vi "MB Serial Example Slave.vi"() -> ()   [LabVIEW 2011]
uses:
  MB Slave Init (poly).vi
  MB Globals.vi
  MB Slave Read All Coils (poly).vi
  MB Slave Read All Holding Registers (poly).vi
  MB Slave Write Input Registers (poly).vi
  MB Slave Write Discrete Inputs (poly).vi
panel:
  in  "VISA resource name":refnum<visa-resource-name>
  in  "Slave Address":u8=1 format="%.0x"
  in  "Timeouts":u32[](array[numeric])=[10000]
  in  "Modes":enum16{"RTU", "ASCII"}[](array[ring])=[enum."RTU"]
  in  "Stop":bool
  out "Holding Registers":u16[](array[numeric]) caption="Holding Registers (Master can write in these registers)"
  out "Coils":bool[](array[boolean]) caption="Coils (Master can write coils)"
  in  "Discrete Inputs":bool[](array[boolean])=[FALSE, FALSE, FALSE, FALSE] caption="Discrete Inputs (Master can only read them)"
  in  "Input Registers":u16[](array[numeric])=[0, 0, 0, 0] caption="Input Registers (Master can only read them)"
  # "MB Serial Example Slave.vi\n\nInstructions\n1. Connect your 2 COMs ports using a cross-over cable\n2. Select a COM port in VISA resouce name\n3. Run the VI\n4. Open and run MB Example Master.vi\n5. Modify the discrete inputs or input registers on the slave -> they're updated on the master.\n6. Modify the coils and registers on the master -> they're updated on the slave."
  # "Serial Settings (Other settings imported from MAX)"
  # "Slave Registers"
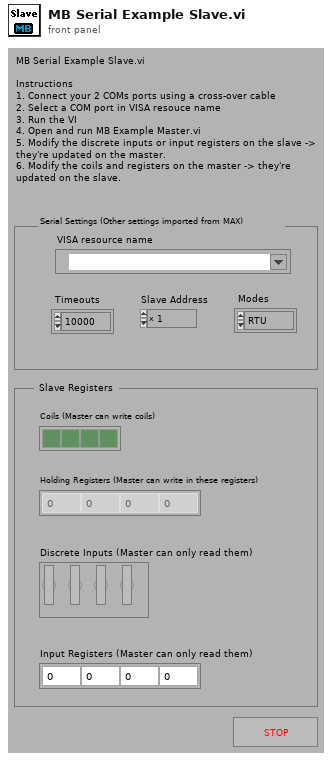
[diagram p1: front panel]
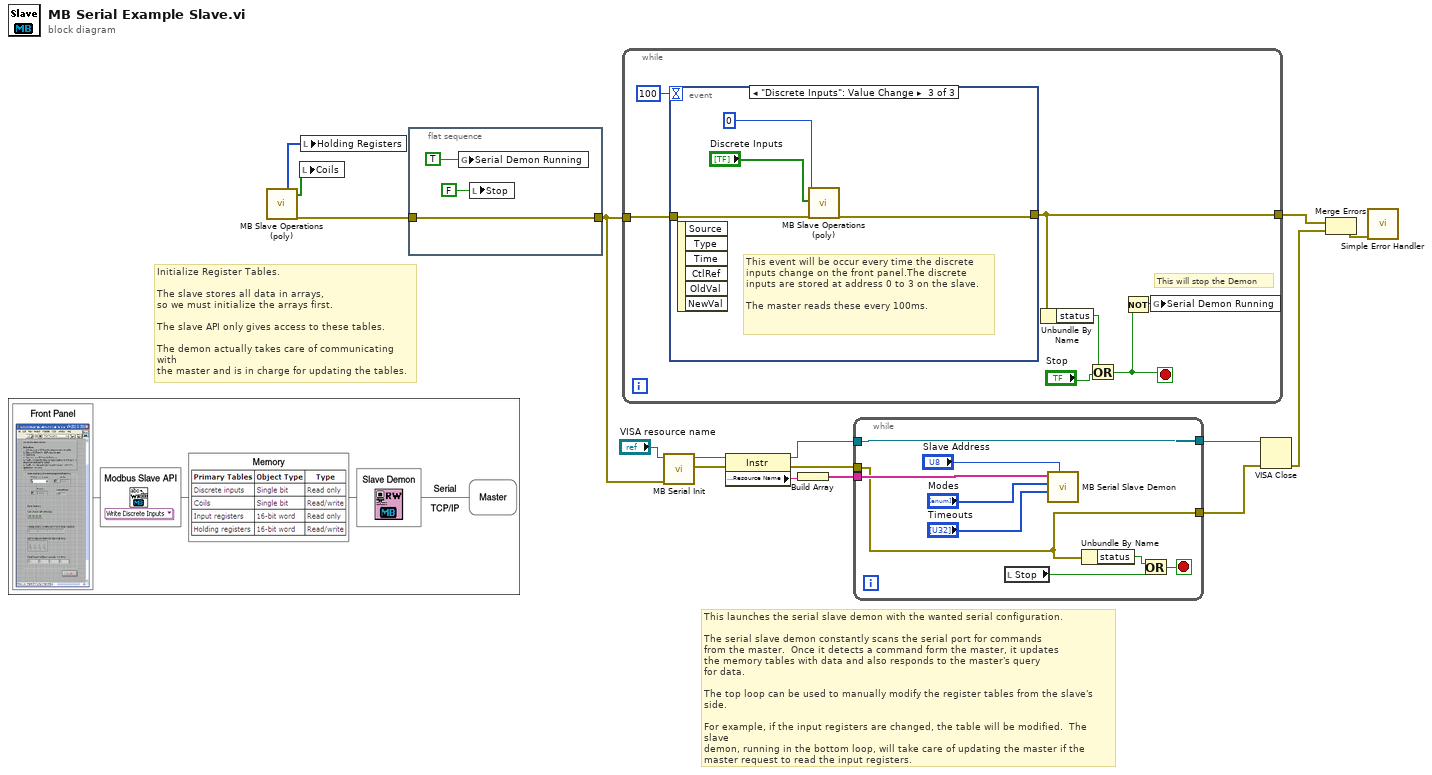
[diagram p0: block diagram]
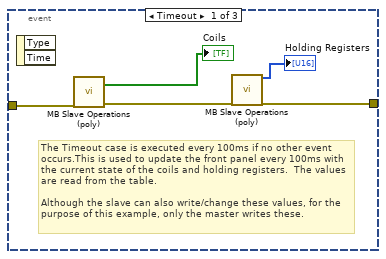
[diagram p2: hidden frame]
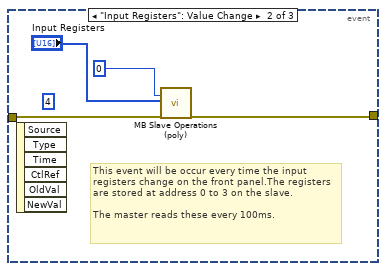
[diagram p3: hidden frame]
diagram:
  # "Initialize Register Tables.\n\nThe slave stores all data in arrays,\nso we must initialize the arrays first.  \n\nThe slave API only gives access to these tables. \n\nThe demon actually takes care of communicating with \nthe master and is in charge for updating the tables."
  # "This launches the serial slave demon with the wanted serial configuration.\n\nThe serial slave demon constantly scans the serial port for commands \nfrom the master.  Once it detects a command form the master, it updates\nthe memory tables with data and also responds to the master's query\nfor data.\n\nThe top loop can be used to manually modify the register tables from the slave's side.\n\nFor example, if the input registers are changed, the table will be modified.  The slave\ndemon, running in the bottom loop, will take care of updating the master if the \nmaster request to read the input registers."
  n1 = call-poly "MB Slave Operations (poly).vi"() -> ("Holding Registers"=w14:u16[], "Coils"=w13:bool[], "error out"=w15:errorcluster)  [unwired: 1 in, 16 out]
  n2 = local write "Coils"(w13) -> ()
  n3 = local write "Holding Registers"(w14) -> ()
  n4 = flat-sequence {
    tunnel: [w18] -> w5
    tunnel: w15 -> [w18]
    frame #0 {
      n5 = global write "MB Globals.vi" "Serial Demon Running"(TRUE ("Slave Demon Running")) -> ()
      n6 = local write "Stop"(FALSE ("Stop")) -> ()
    }
  }
  n7 = while {
    tunnel: w5 -> [w26]
    tunnel: [w22] -> w3
    stop <- w20 stop-if-true
    # "This will stop the Demon"
    n8 = event shown="[2] \"Discrete Inputs\": Value Change" {
      selector: _ -> [_ _ _]
      dyn-events: _ -> [_ _ _]
      timeout: 100 -> [_ _ _]
      tunnel: w26 -> [w31 w35 w39]
      tunnel: [w28 w32 w36] -> w22
      event Timeout {
        # "The Timeout case is executed every 100ms if no other event occurs.This is used to update the front panel every 100ms with the current state of the coils and holding registers.  The values are read from the table. \n\nAlthough the slave can also write/change these values, for the purpose of this example, only the master writes these."
        n9 = event-data() -> ()  [unwired: 3 out]
        n10 = call-poly "MB Slave Operations (poly).vi"("error in"=w31) -> ("Coils"=→"Coils":bool[], "error out"=w29:errorcluster)  [unwired: 17 out]
        n11 = call-poly "MB Slave Operations (poly).vi"("error in"=w29) -> ("Holding Registers"=→"Holding Registers":u16[], "error out"=w28:errorcluster)  [unwired: 17 out]
      }
      event "Input Registers": Value Change {
        (unwired) u16 4 ("Quantity")
        # "This event will be occur every time the input registers change on the front panel.The registers are stored at address 0 to 3 on the slave.\n \nThe master reads these every 100ms."
        n12 = event-data() -> ()  [unwired: 7 out]
        n13 = call-poly "MB Slave Operations (poly).vi"("Starting Address"=u16 0 ("Address"), "Input Registers"="Input Registers", "error in"=w35) -> ("error out"=w32:errorcluster)  [unwired: 1 in, 15 out]
      }
      event "Discrete Inputs": Value Change {
        # "This event will be occur every time the discrete inputs change on the front panel.The discrete inputs are stored at address 0 to 3 on the slave.\n \nThe master reads these every 100ms."
        n14 = event-data() -> ()  [unwired: 7 out]
        n15 = call-poly "MB Slave Operations (poly).vi"("Starting Address"=u16 0, "Discrete Inputs"="Discrete Inputs", "error in"=w39) -> ("error out"=w36:errorcluster)  [unwired: 1 in, 15 out]
      }
    }
    n16 = Unbundle By Name(w22) -> ("status"=w24:bool)
    n17 = Or(x=w24, y="Stop") -> (x .or. y?=w20:bool)
    n18 = Not(x=w20) -> (.not. x?=w21:bool)
    n19 = global write "MB Globals.vi" "Serial Demon Running"(w21) -> ()
  }
  n20 = call "MB Serial Init.vi"("error in (no error)"=w5, "VISA resource name"="VISA resource name") -> ("error out"=w10:errorcluster, "VISA resource name out"=w11:refnum<visa-resource-name>)  [unwired: 5 in, 3 out]
  n21 = property class="Instr"(reference=w11, error in=w10) -> (reference out=w8:refnum<visa-resource-name>, error out=w6:errorcluster, "General Settings:Resource Name"=w9:string)
  n22 = Build Array(w9) -> (w7:string[])
  n23 = while {
    tunnel: [w43] -> w16
    tunnel: w8 -> [w43]
    tunnel: w7 -> [w42]
    tunnel: w6 -> [w41]
    tunnel: [w41] -> w4
    stop <- w44 stop-if-true
    n24 = local read "Stop"() -> (w40:bool)
    n25 = call "MB Serial Slave Demon.vi"("Slave Address"="Slave Address", "Timeouts"="Timeouts", "Modes"="Modes", "VISA Sessions"=w42) -> ()  [unwired: 1 in, 7 out]
    n26 = Unbundle By Name(w41) -> ("status"=w45:bool)
    n27 = Or(x=w45, y=w40) -> (x .or. y?=w44:bool)
  }
  n28 = VISA Close(VISA resource name=w16, error in (no error)=w4) -> (error out=w2:errorcluster)
  n29 = Merge Errors(w3, w2) -> (w1:errorcluster)
  n30 = call <vilib>:"Simple Error Handler.vi"("error in (no error)"=w1) -> ()  [unwired: 1 in, 8 out]
